vi "Convert Hex to String.vi"(9 "bits per element":i32=4 min=1 max=64, 10 "Hex Values":u8[](array[numeric]) format="%.0x") -> (3 "Output String":string)   [LabVIEW 2011]
panel:
  out "Array 2":bool[][](array[boolean])
  out "Array":i32[](array[numeric])
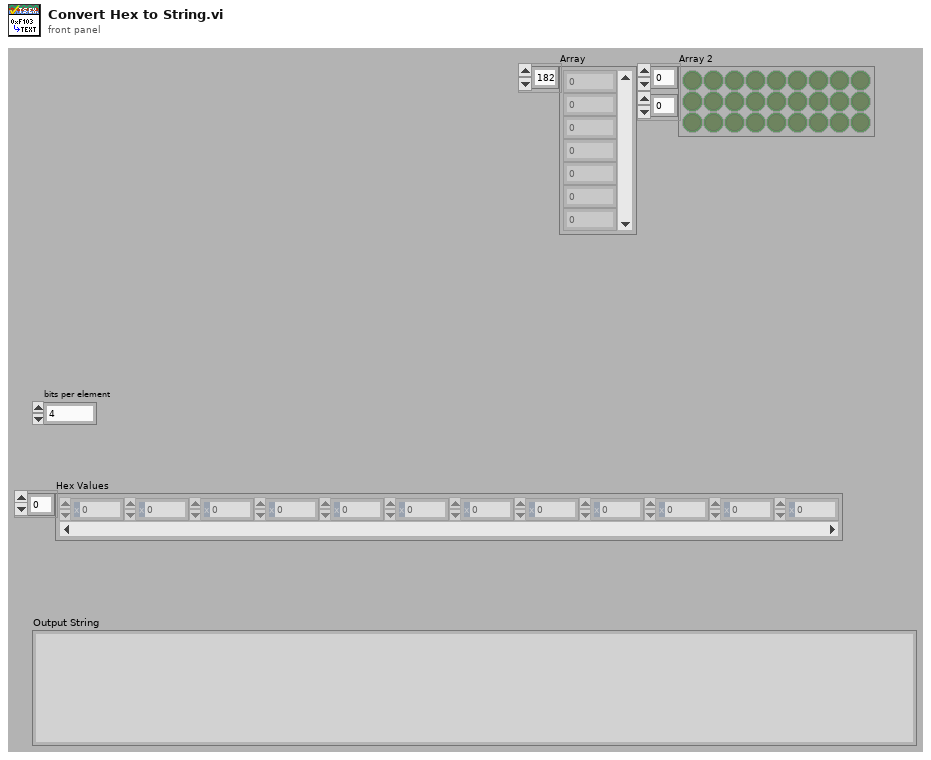
[diagram p1: front panel]
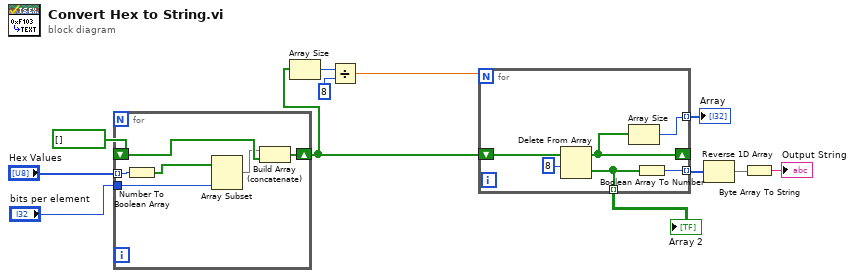
[diagram p0: block diagram]
diagram:
  n1 = for {
    tunnel: "bits per element" -> [w14]
    shift-right: [w16] -> w9
    shift-left: bool[] [] -> [w18]
    tunnel: "Hex Values" -> [w17] mode=indexing
    n2 = Number To Boolean Array(number=w17) -> (Boolean array=w13:bool[])
    n3 = Array Subset(array=w13, length=w14) -> (w15:bool[])  [unwired: 1 in]
    n4 = Build Array (concatenate)(w15, w18) -> (w16:bool[])
  }
  n5 = Array Size(array=w9) -> (size(s)=w11:i32)
  n6 = Divide(x=w11, y=8) -> (x/y=w5:dbl)
  n7 = for {
    N: w5 -> [_]
    shift-right: [w20] -> _
    shift-left: w9 -> [w23]
    tunnel: [w24] -> w2 mode=indexing
    tunnel: [w21] -> w6 mode=indexing
    tunnel: [w19] -> w3 mode=indexing
    n8 = Delete From Array(array=w23, length=8) -> (deleted portion=w19:bool[], array with subset deleted=w20:bool[])  [unwired: 1 in]
    n9 = Array Size(array=w20) -> (size(s)=w21:i32)
    n10 = Boolean Array To Number(Boolean array=w19) -> (number=w24:u32)
  }
  "Array" <- w6
  "Array 2" <- w3
  n11 = Reverse 1D Array(array=w2) -> (reversed array=w1:u32[])
  n12 = Byte Array To String(unsigned byte array=w1) -> (string=→"Output String":string)
